vi "RSZVB Set Automatic Level Control State.vi"(8 "error in (no error)":errorcluster {"code" format="%.0x"}, 10 "ALC State (F: Off)":bool, 11 "VISA session":refnum<visa-resource-name>) -> (0 "error out":errorcluster {"code" format="%.0x"}, 3 "dup VISA session":refnum<visa-resource-name>)   [LabVIEW 2011]
doc: "This VI enables or disables the Automatic Level Control for all channels. \n\nRemote-control command(s):\nDIAGnostic:ALC:SETTings[:STATe] ON | OFF"
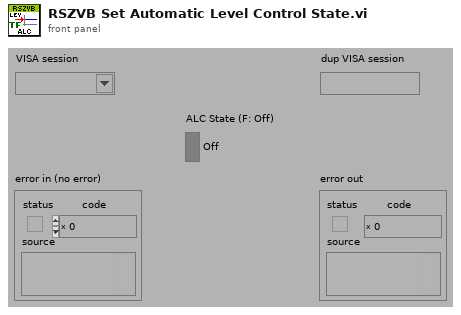
[diagram p1: front panel]
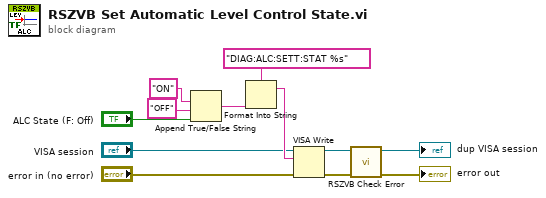
[diagram p0: block diagram]
diagram:
  n1 = Append True/False String(1:"ALC State (F: Off)", 2:"OFF", 3:"ON") -> (0:w6:string)  [unwired: 1 in]
  n2 = Format Into String(format string="DIAG:ALC:SETT:STAT %s", w6) -> (resulting string=w7:string)  [unwired: 2 in, 1 out]
  n3 = VISA Write(VISA resource name="VISA session", write buffer=w7, error in (no error)="error in (no error)") -> (VISA resource name out=w8:refnum<visa-resource-name>, error out=w9:errorcluster)  [unwired: 1 out]
  n4 = call "RSZVB Check Error.vi"("error in (no error)"=w9, "VISA session"=w8) -> ("error out"=→"error out":errorcluster, "dup VISA session"=→"dup VISA session":refnum<visa-resource-name>)  [unwired: 8 in]
